vi "Get MB session in.vi"(11 "EPEVER-MPPT in":refnum<class "EPEVER-MPPT.lvclass">) -> (2 "MB Serial Master:MB_Master":refnum<class "MB_Master.lvclass">, 3 "EPEVER-MPPT out":refnum<class "EPEVER-MPPT.lvclass">)   [LabVIEW 2016, in "EPEVER-MPPT.lvlib" / "EPEVER-MPPT.lvclass"]
uses:
  EPEVER-MPPT.lvclass
  <vilib>/Plasmionique/MB Master/MB_Master/MB_Master.lvclass
  EPEVER-MPPT.lvclass/EPEVER-MPPT.ctl
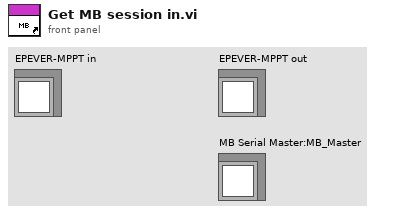
[diagram p1: front panel]
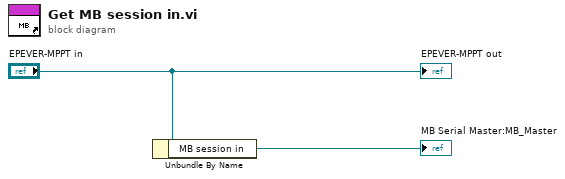
[diagram p0: block diagram]
diagram:
  n1 = Unbundle By Name("EPEVER-MPPT in") -> ("MB session in"=→"MB Serial Master:MB_Master":refnum<class "MB_Master.lvclass">)
  "EPEVER-MPPT out" <- "EPEVER-MPPT in"
